vi "MGCC_StaEst_main_v2.vi"() -> ()   [LabVIEW 2016]
uses:
  Sub-VIs/idx2pha.m
  LabVIEW Data/MathScriptVIs/MCStatic_36913153632_ad7b907c4336c9a4301d4a98ceb40ef6.vi
  Sub-VIs/pha2idx.m
  LabVIEW Data/MathScriptVIs/MCStatic_36913153632_97fc4fd93f18dc21ff9c67b2d181c3f0.vi
  Sub-VIs/zeroinjec.m
  LabVIEW Data/MathScriptVIs/MCStatic_36913153632_38bc0b6d5e7e558b0f110b92ad774f07.vi
  Sub-VIs/cequ.m
  LabVIEW Data/MathScriptVIs/MCStatic_36913153632_190089b8fbd23b5b2e6d7efb94562d92.vi
  Sub-VIs/cjoc.m
  LabVIEW Data/MathScriptVIs/MCStatic_36913153632_76f284c03014805d7ef061346a2ce21b.vi
  Sub-VIs/pnequ.m
  LabVIEW Data/MathScriptVIs/MCStatic_36913153632_51d0ca273e0cdb167781528e825b0617.vi
  Sub-VIs/pnjoc.m
  LabVIEW Data/MathScriptVIs/MCStatic_36913153632_2d91246c5f424d8923cb1d65b269a643.vi
  Sub-VIs/vnequ.m
  LabVIEW Data/MathScriptVIs/MCStatic_36913153632_ab75b36ccfe4f271c5be04de954c4d78.vi
  Sub-VIs/vnjoc.m
  LabVIEW Data/MathScriptVIs/MCStatic_36913153632_e68758472886c7ad71496a2b3f30627d.vi
  <vilib>/imath/engines/lvmath2/RunTimeEngine/IndexRead/NIMS M(S,S).vi
  <vilib>/imath/engines/lvmath2/RunTimeEngine/BuiltInFunctions/abs/NIMS_abs(signed).vi
  <vilib>/imath/engines/lvmath2/RunTimeEngine/RunTimeType/NIMS_RunTimeType_From StrictType (excl LVString).vi
  <vilib>/imath/engines/lvmath2/RunTimeEngine/Struct/NIMS_StructSetField.vi
  <vilib>/imathl/engines/lvmath/Functions/Error Handling/Create Error.vi
  <vilib>/imath/engines/lvmath2/RunTimeEngine/Struct/NIMS_StructGetField.vi
  <vilib>/imath/engines/lvmath2/RunTimeEngine/RunTimeType/NIMS_RunTimeType_To Numeric.vi
  <vilib>/imath/engines/lvmath2/RunTimeEngine/IndexRead/NIMS M($,R2).vi
  <vilib>/imath/engines/lvmath2/RunTimeEngine/BuiltInFunctions/imag/NIMS_imag(Complex).vi
  <vilib>/imath/engines/lvmath2/RunTimeEngine/BuiltInFunctions/angle/NIMS_angle.vi
  <vilib>/imath/engines/lvmath2/RunTimeEngine/VariableToken/Support/NIMS_Matrix Boolean Index to I32 Index.vi
  <vilib>/imath/engines/lvmath2/RunTimeEngine/IndexReplace/NIMS M(V)=S.vi
  <vilib>/imath/engines/lvmath2/RunTimeEngine/BuiltInFunctions/size/NIMS_I32=size(GCol,I32).vi
  <vilib>/imath/engines/lvmath2/RunTimeEngine/RangeToken/NIMS_Range_R2 - Integer.vi
  <vilib>/imath/engines/lvmath2/RunTimeEngine/IndexRead/NIMS V(S).vi
  <vilib>/imath/engines/lvmath2/RunTimeEngine/MatrixToken/NIMS_MatrixToken_M_RV.vi
  <vilib>/imath/engines/lvmath2/RunTimeEngine/ErrorHandling/NIMS_Create Error From Enums.vi
  <vilib>/imath/engines/lvmath2/RunTimeEngine/CommandStatement/MC_CommandStatement_break.vi
  <vilib>/imath/engines/lvmath2/RunTimeEngine/RangeToken/NIMS_Range.vi
  <vilib>/imath/engines/lvmath2/RunTimeEngine/MatrixToken/NIMS_MatrixToken_M_SorCV.vi
  <vilib>/imath/engines/lvmath2/RunTimeEngine/BuiltInFunctions/rand/NIMS_rand(I32,I32).vi
  <vilib>/imath/engines/lvmath2/RunTimeEngine/ErrorHandling/NIMS_Error From Error Code.vi
  <vilib>/imath/engines/lvmath2/RunTimeEngine/ArithmeticOperatorToken/NIMS_ArithmeticOperator_plus.vi
  <vilib>/imath/engines/lvmath/Functions/Error Handling/MergeErrorsWrapper.vi
  <vilib>/imath/engines/lvmath2/RunTimeEngine/ArithmeticOperatorToken/NIMS_ArithmeticOperator_times.vi
  <vilib>/imath/engines/lvmath2/RunTimeEngine/BuiltInFunctions/reshapemx/NIMS_[GV]_reshapemx.vi
  <vilib>/imath/engines/lvmath2/RunTimeEngine/IndexRead/NIMS M(M).vi
  <vilib>/imath/engines/lvmath2/RunTimeSupport/NIMS_Error if Not Equal.vi
  <vilib>/imath/engines/lvmath2/RunTimeEngine/MatrixToken/NIMS_MatrixToken_M_M.vi
  <vilib>/imath/engines/lvmath2/RunTimeEngine/IndexRead/NIMS M($,S).vi
  <vilib>/imath/engines/lvmath2/RunTimeEngine/BuiltInFunctions/size/NIMS_I32Row=size(GM).vi
  <vilib>/imath/engines/lvmath2/RunTimeEngine/BuiltInFunctions/ones/NIMS_M=ones(I32V).vi
  <vilib>/imath/engines/lvmath2/RunTimeEngine/BuiltInFunctions/diag/NIMS_diag.vi
  <vilib>/imath/engines/lvmath2/RunTimeEngine/RowToken/NIMS_RowToken_CV_CV.vi
  <vilib>/imath/engines/lvmath2/RunTimeEngine/BuiltInFunctions/zeros/NIMS_M=zeros(I32,I32).vi
  <vilib>/imath/engines/lvmath2/RunTimeEngine/RangeToken/NIMS_Range_R2 - Float.vi
  <vilib>/imath/engines/lvmath2/RunTimeEngine/IndexReplace/NIMS M(S,S)=S.vi
  <vilib>/imath/engines/lvmath2/RunTimeEngine/IndexReplace/NIMS M($,V)=S.vi
  <vilib>/imath/engines/lvmath2/RunTimeEngine/ArithmeticOperatorToken/NIMS_ArithmeticOperator_minus.vi
  <vilib>/imath/engines/lvmath2/RunTimeEngine/ArithmeticOperatorToken/NIMS_ArithmeticOperator_rightdivmx.vi
  <vilib>/imath/engines/lvmath2/RunTimeEngine/ArithmeticOperatorToken/NIMS_ArithmeticOperator_multmx(M,CV).vi
  <vilib>/imath/engines/lvmath2/RunTimeEngine/ArithmeticOperatorToken/NIMS_ArithmeticOperator_multmx.vi
  <vilib>/imath/engines/lvmath2/RunTimeEngine/BuiltInFunctions/pinv/NIMS_pinv.vi
  <vilib>/imath/engines/lvmath2/RunTimeEngine/BuiltInFunctions/max/1 input/NIMS_max(RM).vi
  <vilib>/imath/engines/lvmath2/RunTimeEngine/IndexRead/NIMS M(V).vi
  <vilib>/imath/engines/lvmath2/RunTimeEngine/BuiltInFunctions/reshapemx/NIMS_[GM]_reshapemx.vi
  <vilib>/imath/engines/lvmath2/RunTimeEngine/VariableToken/NIMS_VariableToken_CondDefined.vi
  <vilib>/imath/engines/lvmath2/RunTimeEngine/NodeEndStatement/NIMS_NodeEndStatement_Output.vi
  <vilib>/imath/engines/lvmath2/RunTimeEngine/ErrorHandling/NIMS_Finalize Error.vi
  <instcachedir>/0/MCStatic_36913153632_190089b8fbd23b5b2e6d7efb94562d92_04760DF2195B45A9A1E78E905702ACD7.lvgen/MCStatic_36913153632_190089b8fbd23b5b2e6d7efb94562d92_04760DF2195B45A9A1E78E905702ACD7_000.vi
  <instcachedir>/0/MCStatic_36913153632_190089b8fbd23b5b2e6d7efb94562d92_04760DF2195B45A9A1E78E905702ACD7.lvgen/MCStatic_36913153632_190089b8fbd23b5b2e6d7efb94562d92_04760DF2195B45A9A1E78E905702ACD7_001.vi
  <instcachedir>/0/MCStatic_36913153632_2d91246c5f424d8923cb1d65b269a643_99EB49824A304C41840E98C0AACBDA94.lvgen/MCStatic_36913153632_2d91246c5f424d8923cb1d65b269a643_99EB49824A304C41840E98C0AACBDA94_000.vi
  <instcachedir>/0/MCStatic_36913153632_2d91246c5f424d8923cb1d65b269a643_99EB49824A304C41840E98C0AACBDA94.lvgen/MCStatic_36913153632_2d91246c5f424d8923cb1d65b269a643_99EB49824A304C41840E98C0AACBDA94_001.vi
  <instcachedir>/0/MCStatic_36913153632_38bc0b6d5e7e558b0f110b92ad774f07_C6B76AB5891B40F4803FB2B48654B2A9.lvgen/MCStatic_36913153632_38bc0b6d5e7e558b0f110b92ad774f07_C6B76AB5891B40F4803FB2B48654B2A9_000.vi
  <instcachedir>/0/MCStatic_36913153632_51d0ca273e0cdb167781528e825b0617_78BD2D51507D495384DAB15CC2E74117.lvgen/MCStatic_36913153632_51d0ca273e0cdb167781528e825b0617_78BD2D51507D495384DAB15CC2E74117_000.vi
  <instcachedir>/0/MCStatic_36913153632_51d0ca273e0cdb167781528e825b0617_78BD2D51507D495384DAB15CC2E74117.lvgen/MCStatic_36913153632_51d0ca273e0cdb167781528e825b0617_78BD2D51507D495384DAB15CC2E74117_001.vi
  <instcachedir>/0/MCStatic_36913153632_76f284c03014805d7ef061346a2ce21b_467DC59D703B4C059BCE920F73FB777B.lvgen/MCStatic_36913153632_76f284c03014805d7ef061346a2ce21b_467DC59D703B4C059BCE920F73FB777B_000.vi
  <instcachedir>/0/MCStatic_36913153632_97fc4fd93f18dc21ff9c67b2d181c3f0_5C608B65A2894F51BDE53CCFA2671AA2.lvgen/MCStatic_36913153632_97fc4fd93f18dc21ff9c67b2d181c3f0_5C608B65A2894F51BDE53CCFA2671AA2_001.vi
  <instcachedir>/0/MCStatic_36913153632_ab75b36ccfe4f271c5be04de954c4d78_5415EF0E754840E594AB8FD8AC33B8AD.lvgen/MCStatic_36913153632_ab75b36ccfe4f271c5be04de954c4d78_5415EF0E754840E594AB8FD8AC33B8AD_000.vi
  <instcachedir>/0/MCStatic_36913153632_ab75b36ccfe4f271c5be04de954c4d78_5415EF0E754840E594AB8FD8AC33B8AD.lvgen/MCStatic_36913153632_ab75b36ccfe4f271c5be04de954c4d78_5415EF0E754840E594AB8FD8AC33B8AD_001.vi
  <instcachedir>/0/MCStatic_36913153632_ad7b907c4336c9a4301d4a98ceb40ef6_619BD3C3D0E2458093F45E8BEE83E1A2.lvgen/MCStatic_36913153632_ad7b907c4336c9a4301d4a98ceb40ef6_619BD3C3D0E2458093F45E8BEE83E1A2_001.vi
  <instcachedir>/0/MCStatic_36913153632_e68758472886c7ad71496a2b3f30627d_43D178B5FAE045E8B9BC672F6734B959.lvgen/MCStatic_36913153632_e68758472886c7ad71496a2b3f30627d_43D178B5FAE045E8B9BC672F6734B959_000.vi
  <instcachedir>/0/MCStatic_36913153632_e68758472886c7ad71496a2b3f30627d_43D178B5FAE045E8B9BC672F6734B959.lvgen/MCStatic_36913153632_e68758472886c7ad71496a2b3f30627d_43D178B5FAE045E8B9BC672F6734B959_001.vi
panel:
  out "index":i32
  out "puTrue":T1
  out "Num":T2
  out "Loc":cluster{"Zeroinj":i32[][], "Line":dbl[][]}
  out "seResult":T3
  out "str_MGCC_MdlMgmt_Feeder":T4
  out "error out":errorcluster
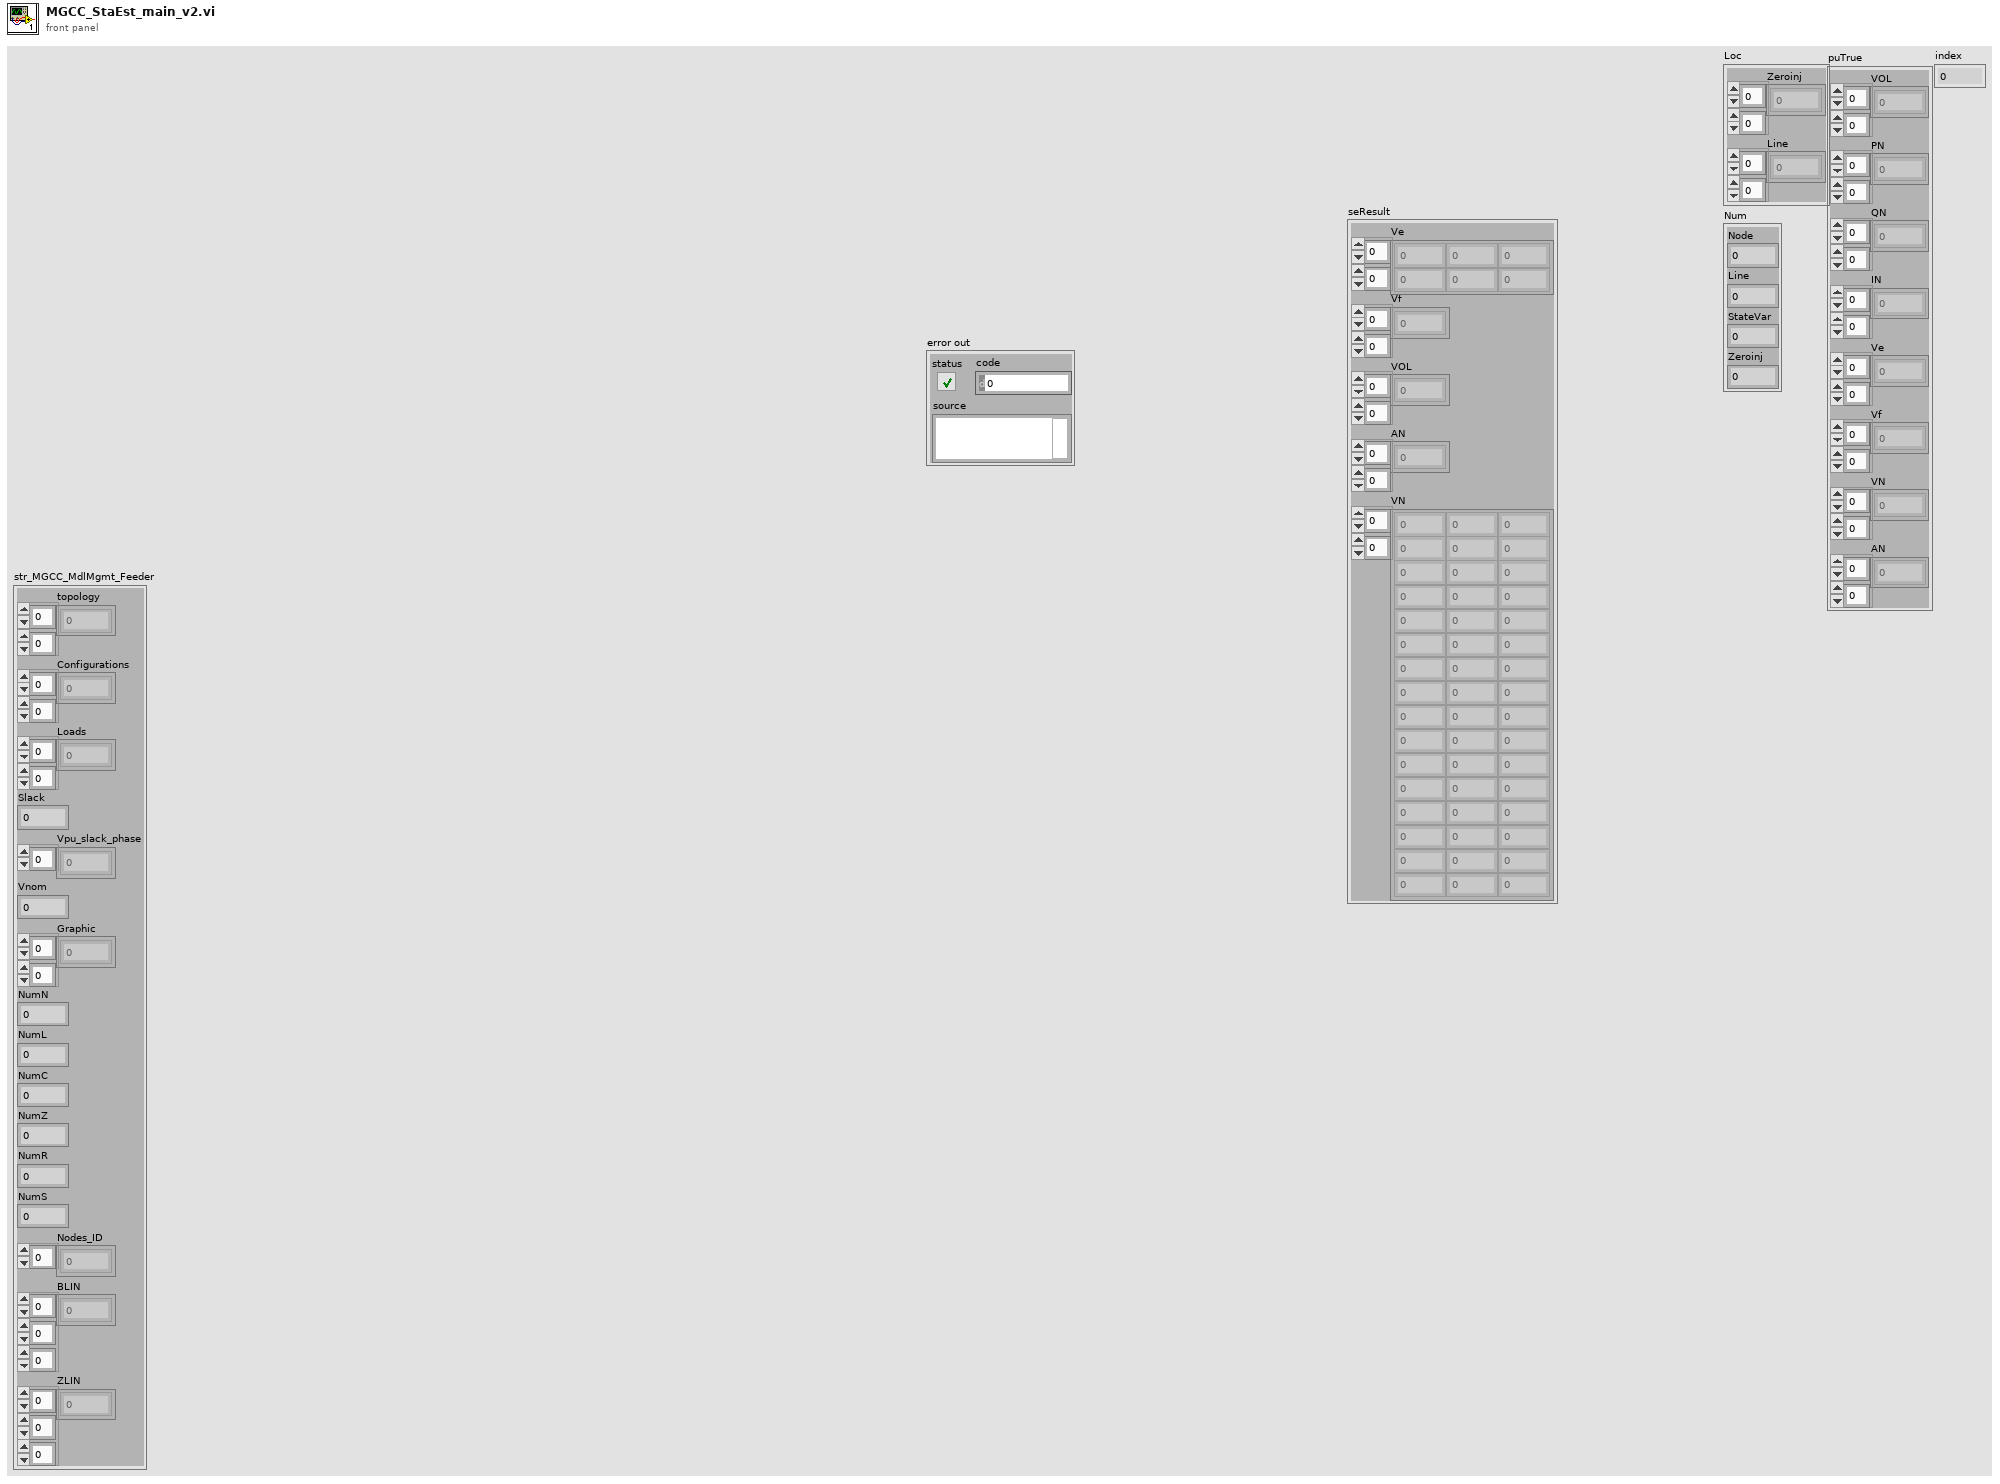
[diagram p1: front panel]
types:
  T1 = cluster{"VOL":cdb[][], "PN":dbl[][], "QN":dbl[][], "IN":dbl[][], "Ve":dbl[][], "Vf":dbl[][], "VN":dbl[][], "AN":dbl[][]}
  T2 = cluster{"Node":dbl, "Line":dbl, "StateVar":i32, "Zeroinj":i32}
  T3 = cluster{"Ve":dbl[][], "Vf":dbl[][], "VOL":cdb[][], "AN":dbl[][], "VN":dbl[][]}
  T4 = cluster{"topology":dbl[][], "Configurations":dbl[][], "Loads":dbl[][], "Slack":dbl, "Vpu_slack_phase":cdb[], "Vnom":dbl, "Graphic":dbl[][], "NumN":dbl, "NumL":dbl, "NumC":dbl, "NumZ":dbl, "NumR":dbl, "NumS":dbl, "Nodes_ID":dbl[], "BLIN":cdb[][][], "ZLIN":cdb[][][]}
  T5 = cluster{"PN":dbl[][], "QN":dbl[][], "VN":dbl[][]}
  T6 = cluster{"Sbase":dbl, "Vbase":dbl, "Ibase":dbl, "Ybase":dbl}
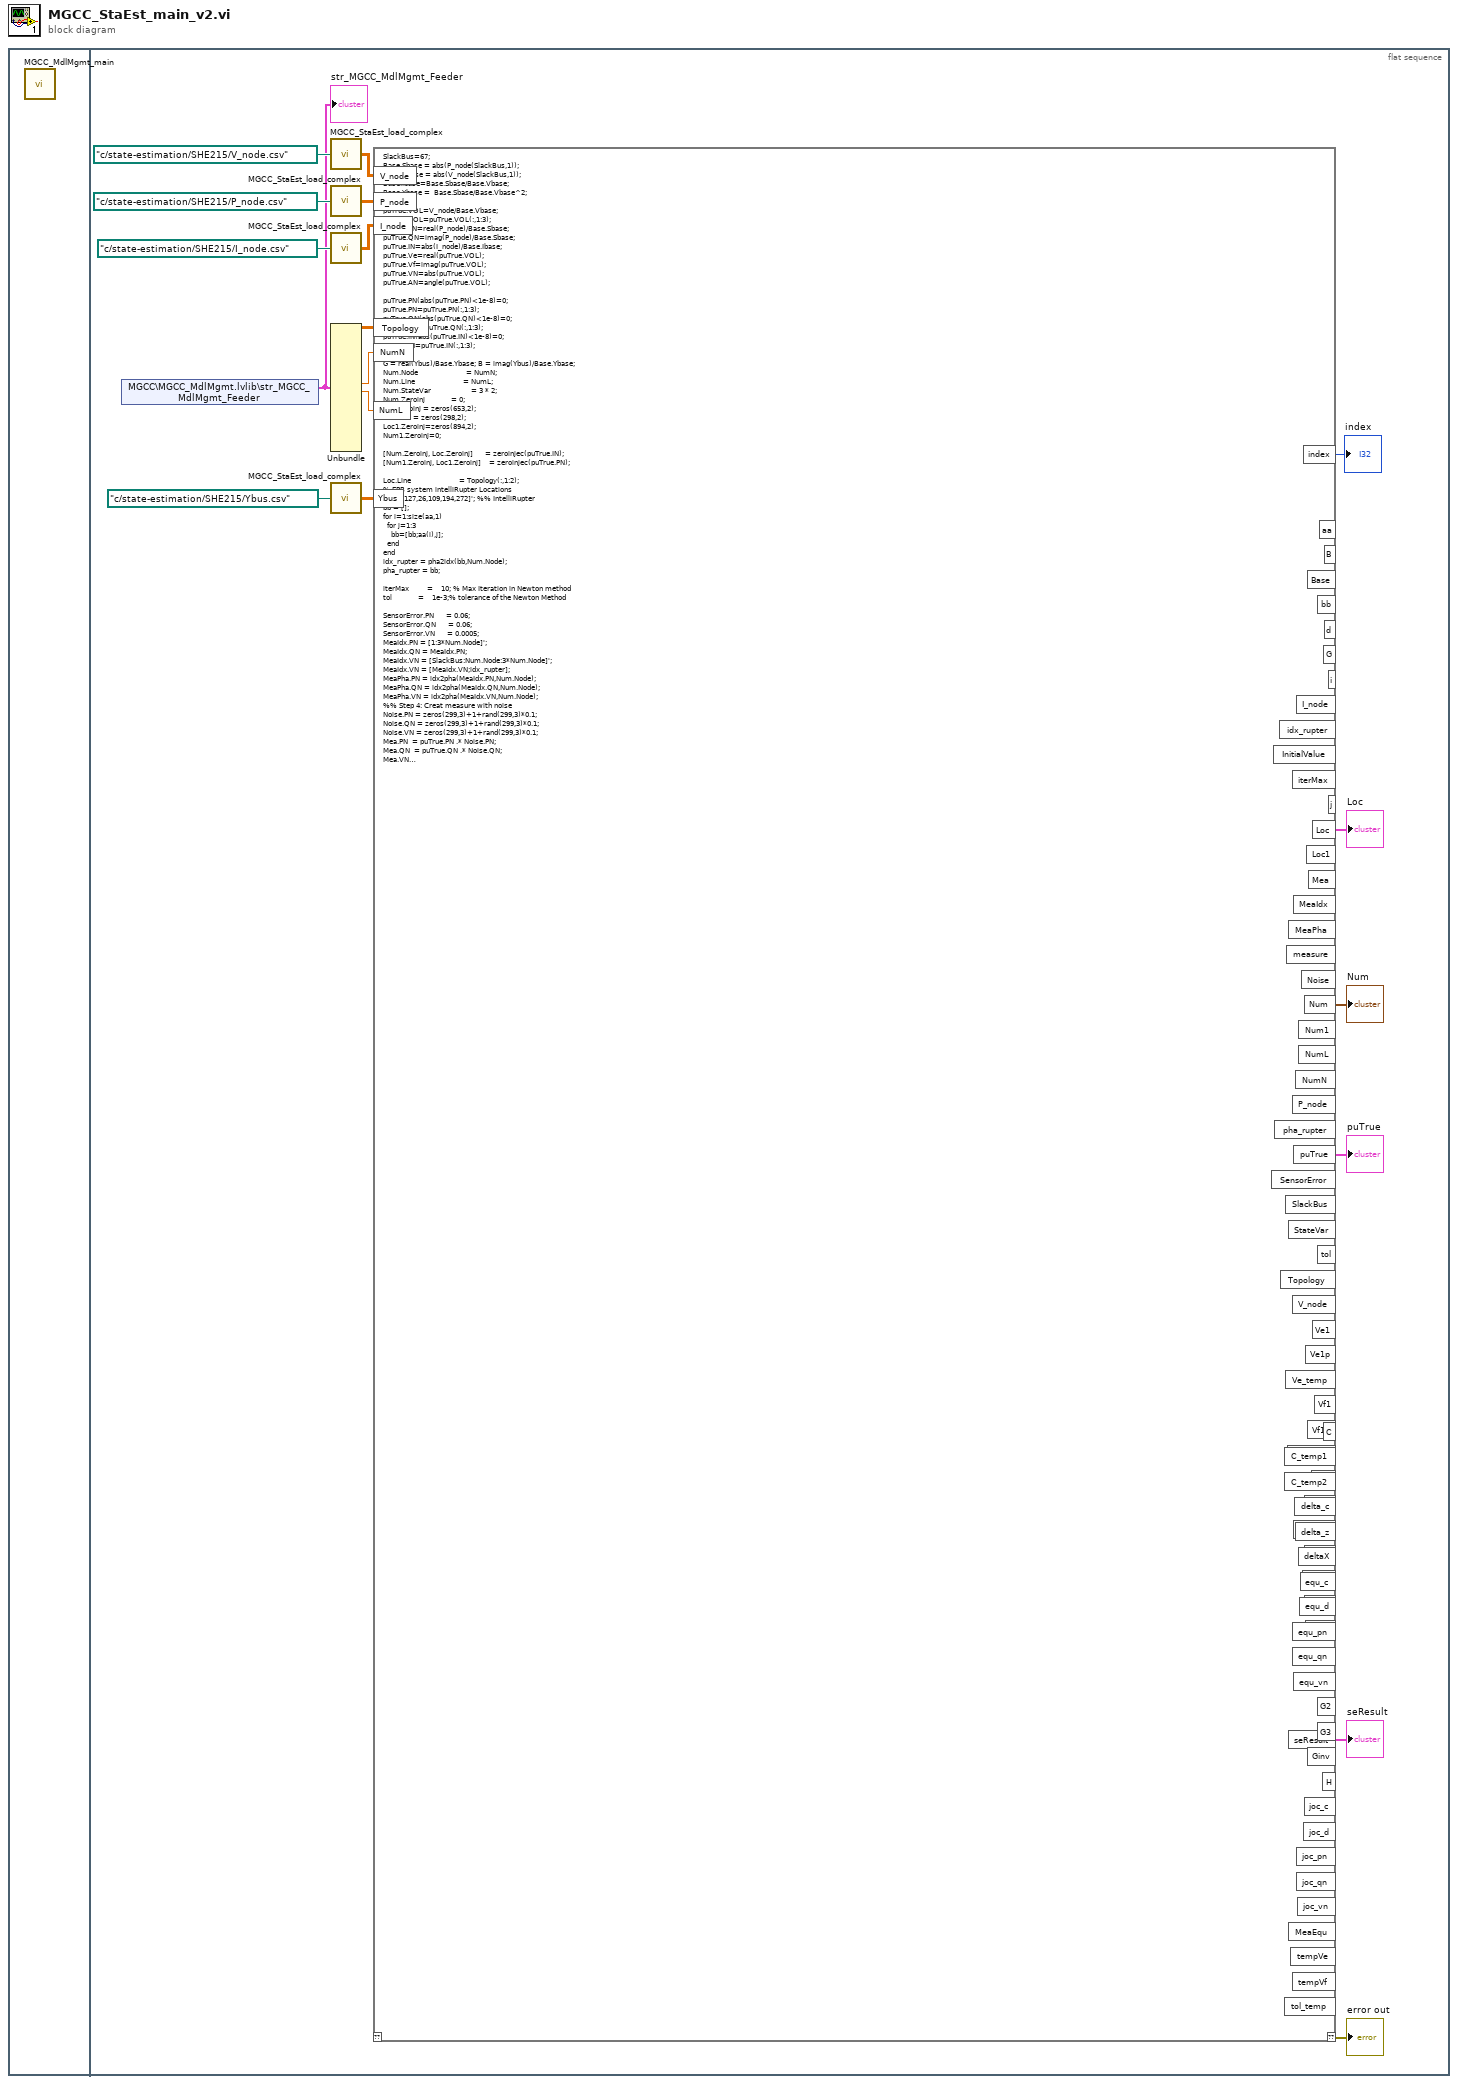
[diagram p0: block diagram]
diagram:
  n1 = flat-sequence {
    frame #0 {
      n2 = call "MGCC_MdlMgmt_main.vi"() -> ()  [unwired: 12 in]
    }
    frame #1 {
      n3 = shared-variable "MGCC\\MGCC_MdlMgmt.lvlib\\str_MGCC_MdlMgmt_Feeder"() -> (w11:T4)  [unwired: 1 in, 1 out]
      "str_MGCC_MdlMgmt_Feeder" <- w11
      n4 = call "MGCC_StaEst_load_complex.vi"("file path (dialog if empty)"=path "c:/state-estimation/SHE215/V_node.csv" ("file path (use dialog)")) -> ("Array 13"=w14:cdb[][])
      n5 = call "MGCC_StaEst_load_complex.vi"("file path (dialog if empty)"=path "c:/state-estimation/SHE215/P_node.csv" ("file path (use dialog)")) -> ("Array 13"=w13:cdb[][])
      n6 = call "MGCC_StaEst_load_complex.vi"("file path (dialog if empty)"=path "c:/state-estimation/SHE215/I_node.csv" ("file path (use dialog)")) -> ("Array 13"=w12:cdb[][])
      n7 = Unbundle(w11) -> ("topology"=w6:dbl[][], "NumN"=w10:dbl, "NumL"=w9:dbl)  [unwired: 13 out]
      n8 = call "MGCC_StaEst_load_complex.vi"("file path (dialog if empty)"=path "c:/state-estimation/SHE215/Ybus.csv" ("file path (use dialog)")) -> ("Array 13"=w7:cdb[][])
      n9 = mathscript code="SlackBus=67;\nBase.Sbase = abs(P_node(SlackBus,1));\nBase.Vbase = abs(V_node(SlackBus,1));\nBase.Ibase=Base.Sbase/Base.Vbase;\nBase.Ybase =  Base.Sbase/Base.Vbase^2;\n\npuTrue.VOL=V_node/Base.Vbase;\npuTrue.VOL=puTrue.VOL(:,1:3);\npuTrue.PN=real(P_node)/Base.Sbase;\npuTrue.QN=imag(P_node)/Base.Sbase;\npuTrue.IN=abs(I_node)/Base.Ibase;\npuTrue.Ve=real(puTrue.VOL);\npuTrue.Vf=imag(puTrue.VOL); \npuTrue.VN=abs(puTrue.VOL);\npuTrue.AN=angle(puTrue.VOL);\n\npuTrue.PN(abs(puTrue.PN)<1e-8)=0;\npuTrue.PN=puTrue.PN(:,1:3);\npuTrue.QN(abs(puTrue.QN)<1e-8)=0;\npuTrue.QN=puTrue.QN(:,1:3);\npuTrue.IN(abs(puTrue.IN)<1e-8)=0;\npuTrue.IN=puTrue.IN(:,1:3);\n\nG = real(Ybus)/Base.Ybase; B = imag(Ybus)/Base.Ybase;\nNum.Node                        = NumN;\nNum.Line                        = NumL;\nNum.StateVar                    = 3 * 2;  \nNum.Zeroinj             = 0;\nLoc.Zeroinj = zeros(653,2);\nLoc.Line = zeros(298,2);\nLoc1.Zeroinj=zeros(894,2);\nNum1.Zeroinj=0;\n\n[Num.Zeroinj, Loc.Zeroinj]      = zeroinjec(puTrue.IN);\n[Num1.Zeroinj, Loc1.Zeroinj]    = zeroinjec(puTrue.PN);\n\nLoc.Line                        = Topology(:,1:2);\n% EPB system intelliRupter Locations\naa = [127,26,109,194,272]'; %% IntelliRupter\nbb = [];\nfor i=1:size(aa,1)\n  for j=1:3\n    bb=[bb;aa(i),j];\n  end\nend\nidx_rupter = pha2idx(bb,Num.Node);\npha_rupter = bb;\n\niterMax         =    10; % Max Iteration in Newton method\ntol             =    1e-3;% tolerance of the Newton Method\n\nSensorError.PN      = 0.06;\nSensorError.QN      = 0.06;\nSensorError.VN      = 0.0005;\nMeaIdx.PN = [1:3*Num.Node]';\nMeaIdx.QN = MeaIdx.PN;\nMeaIdx.VN = [SlackBus:Num.Node:3*Num.Node]';\nMeaIdx.VN = [MeaIdx.VN;idx_rupter]; \nMeaPha.PN = idx2pha(MeaIdx.PN,Num.Node);\nMeaPha.QN = idx2pha(MeaIdx.QN,Num.Node);\nMeaPha.VN = idx2pha(MeaIdx.VN,Num.Node);\n%% Step 4: Creat measure with noise\nNoise.PN = zeros(299,3)+1+rand(299,3)*0.1;\nNoise.QN = zeros(299,3)+1+rand(299,3)*0.1;\nNoise.VN = zeros(299,3)+1+rand(299,3)*0.1;\nMea.PN  = puTrue.PN .* Noise.PN; \nMea.QN  = puTrue.QN .* Noise.QN;\nMea.VN  = puTrue.VN.^2 .* Noise.VN;\nMea.PN  = reshape(Mea.PN,3*Num.Node,1);\nMea.QN  = reshape(Mea.QN,3*Num.Node,1);\nMea.VN  = reshape(Mea.VN,3*Num.Node,1);\nmeasure = [Mea.PN(MeaIdx.PN); Mea.QN(MeaIdx.QN);Mea.VN(MeaIdx.VN)];\nmeasure = measure(:,1);\n\nWPN = SensorError.PN*ones(size(MeaIdx.PN));\nWQN = SensorError.QN*ones(size(MeaIdx.QN));\nWVN = SensorError.VN*ones(size(MeaIdx.VN));\n\nWeight =diag([WPN.^2;WQN.^2;WVN.^2]);\n\nVe1 = reshape(puTrue.Ve,3*Num.Node,1);\nVf1 = reshape(puTrue.Vf,3*Num.Node,1);\nVV1 = [Ve1,Vf1];\nStateVar= reshape(VV1',Num.StateVar * Num.Node,1);\n       \nVe_temp = zeros(Num.Node,3);\nVf_temp = zeros(Num.Node,3);\n\nfor i=1:Num.Node\n    for d=1:3\n        if puTrue.Ve(i,d) == 0\n            Ve_temp(i,d)=0;Vf_temp(i,d)=0;\n        else\n            if d==1\n                Ve_temp(i,d)=0.989*cos(-33.49*pi/180);\n                Vf_temp(i,d)=-0.989*sin(-33.49*pi/180);\n            end\n            if d==2\n                Ve_temp(i,d)=0.993*cos(-153.64*pi/180);\n                Vf_temp(i,d)=-0.993*sin(-153.64*pi/180);\n            end\n            if d==3\n                Ve_temp(i,d)=0.99*cos(86.14*pi/180);\n                Vf_temp(i,d)=-0.99*sin(86.14*pi/180);            \n            end\n        end\n    end\nend\n\nVe1p = reshape(Ve_temp,3*Num.Node,1);\nVf1p = reshape(Vf_temp,3*Num.Node,1);\nVV1p = [Ve1p,-Vf1p];\nInitialValue = reshape(VV1p',Num.StateVar*Num.Node,1);\n\n\nfor i = 1:iterMax\n  % Jocobian matrix\n  [joc_pn,joc_qn] = pnjoc(Num,StateVar,MeaPha,B,G);\n  joc_vn          = vnjoc(Num,StateVar,MeaPha);\n  H = [joc_pn;joc_qn;joc_vn];\n  H(:,2*SlackBus:2*Num.Node:end)=0;   \n  H(:,2*SlackBus-1:2*Num.Node:end)=0; \nindex=i;\n  % MeaEqu\n  [equ_pn,equ_qn] = pnequ(Num,StateVar,MeaPha,B,G);\n  equ_vn = vnequ(Num,StateVar,MeaPha);\n  MeaEqu = [equ_pn;equ_qn;equ_vn];\n  \n  delta_z = measure-MeaEqu;\n  G2 = H'/Weight*delta_z;\n  G3 = H'/Weight*H;    \n  Ginv = pinv(G3);\n  \n  [joc_c,joc_d] = cjoc(Num,B,G,Loc);\n  C = [joc_c;joc_d];\n  C(:,2*SlackBus:2*Num.Node:end)=0;\n  C(:,2*SlackBus-1:2*Num.Node:end)=0;\n  [equ_c,equ_d] = cequ(Num,StateVar,B,G,Loc);\n  delta_c = [-equ_c;-equ_d];  \n  C_temp1 = C*Ginv*C';\n  C_temp2 = pinv(C_temp1);\n  deltaX = Ginv * G2 -Ginv*C'*(C_temp2*(C*Ginv*G2-delta_c)); \n\n  deltaX(abs(deltaX)<1e-8)=0;\n  tol_temp = max(abs(deltaX));\n  if tol_temp < tol\n      break;\n  end\n  StateVar = StateVar + deltaX;\nend\n\ntempVe=StateVar(1:2:6*Num.Node-1);\ntempVf=StateVar(2:2:6*Num.Node);\nseResult.Ve=reshape(tempVe,Num.Node,3);\nseResult.Vf=reshape(tempVf,Num.Node,3);\nseResult.VOL=seResult.Ve+1i*seResult.Vf;\nseResult.AN=angle(seResult.VOL);\nseResult.VN=abs(seResult.VOL);"("V_node"=w14, "P_node"=w13, "I_node"=w12, "NumN"=w10, "NumL"=w9, "Ybus"=w7, "Topology"=w6) -> ("??"=→"error out":errorcluster, "seResult"=→"seResult":T3, "Loc"=→"Loc":cluster{"Zeroinj":i32[][], "Line":dbl[][]}, "Num"=→"Num":T2, "puTrue"=→"puTrue":T1, "index"=→"index":i32)  [unwired: 1 in, 66 out]
    }
  }
